vi "Aurora Tx Config.vi"(0 "6592R Resources":T3[](array[typedef]), 7 "FIFO Depth":u32=10240000 format="%#.6p", 11 "error in (no error)":errorcluster, 12 "tx config":T1={"rf enable 0"=FALSE, "rf config 0"={"antenna"="TX1", "frequency"=2000000000.0, "lo frequency"=-1.0, "level"=0.0}, "rf enable 1"=FALSE, "rf config 1"={"antenna"="TX1", "frequency"=2000000000.0, "lo frequency"=-1.0, "level"=0.0}, "transfer mode"=enum."Finite", "sample rate"=10000000.0, "start trigger"=enum."Immediate"} {"sample rate" format="%#.3pS/s"; "rf config 0"."level" format="%#_gdBm"; "rf config 0"."lo frequency" format="%#.3pHz"; "rf config 0"."frequency" format="%#.3pHz"; "rf config 1"."level" format="%#_gdBm"; "rf config 1"."lo frequency" format="%#.3pHz"; "rf config 1"."frequency" format="%#.3pHz"}) -> (4 "Ports used":bool[](array[boolean]), 6 "Refnum out":refnum<k20>[](array[refnum]), 8 "Actual FIFO Depths":u32[][](array[numeric]), 10 "2 Ports?":bool[](array[boolean]), 15 "error out":errorcluster)   [LabVIEW 2016]
uses:
  <vilib>/userdefined/Silver/nirio_resource_slv.ctl
  TypeDefs/Tx Config.ctl
  2954/SubVIs/Start Trigger.ctl
  6592R/SubVIs/Aurora Stream (NI 6592R) (Host).lvlib
panel:
  out "sFrontEndConfig_Complete":bool
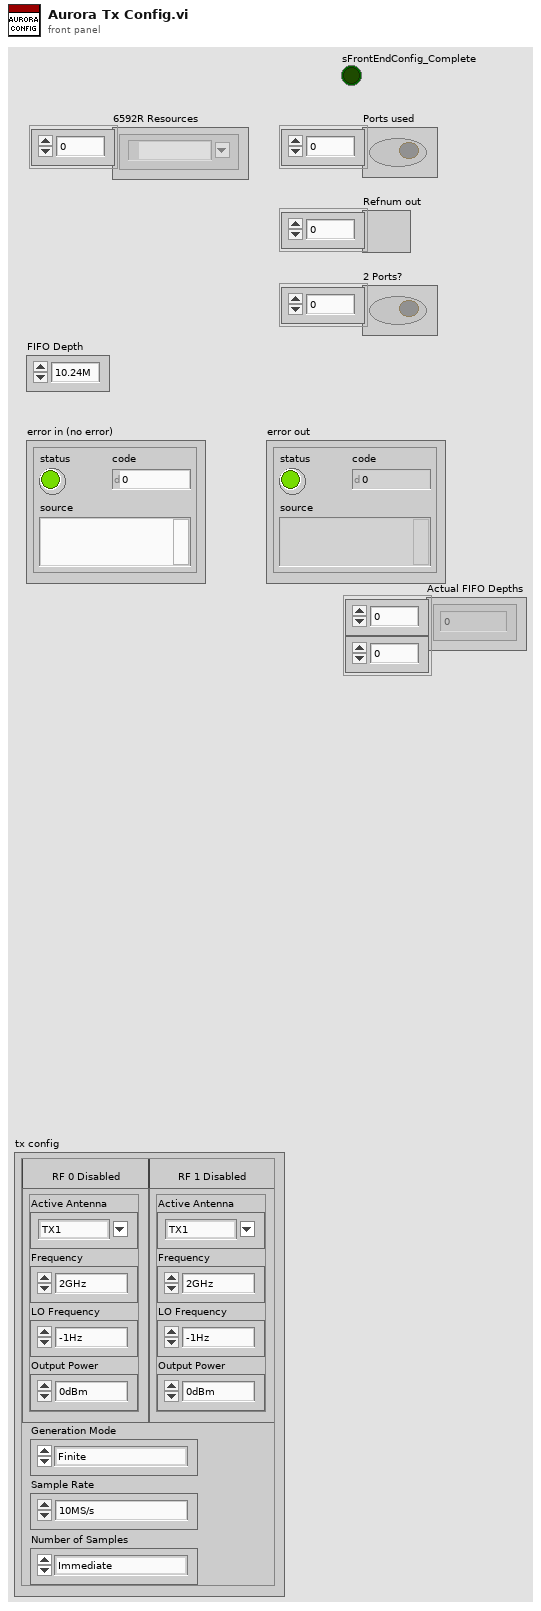
[diagram p1: front panel]
types:
  T1 = typedef "Tx Config.ctl" = cluster{"rf enable 0":bool, "rf config 0":cluster{"antenna":string, "frequency":dbl, "lo frequency":dbl, "level":dbl}, "rf enable 1":bool, "rf config 1":cluster{"antenna":string, "frequency":dbl, "lo frequency":dbl, "level":dbl}, "transfer mode":enum16{"Finite", "Continuous"}, "sample rate":dbl, "start trigger":T2}
  T2 = typedef "Start Trigger.ctl" = enum8{"Software", "Digital Edge", "Rx Start Trigger", "Tx Start Trigger", "Immediate", "Future Time Event"}
  T3 = typedef "nirio_resource_slv.ctl" = tag
  T4 = cluster{"Hard Error":bool, "Soft Error":bool, "Lane Up":bool, "Channel Up":bool, "Sys Reset":bool}
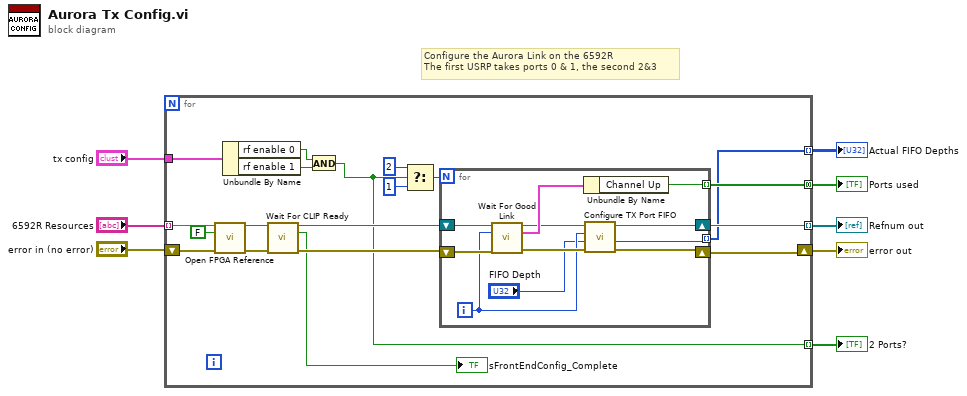
[diagram p0: block diagram]
diagram:
  # "Configure the Aurora Link on the 6592R\nThe first USRP takes ports 0 & 1, the second 2&3"
  n1 = for {
    tunnel: [w20] -> w5 mode=indexing
    tunnel: "6592R Resources" -> [w25] mode=indexing
    shift-right: [w21] -> w4
    shift-left: "error in (no error)" -> [w24]
    tunnel: [w17] -> w8 mode=concatenating
    tunnel: [w14] -> w3 mode=indexing
    tunnel: "tx config" -> [w13]
    tunnel: [w12] -> w1 mode=indexing
    n2 = call "Open FPGA Reference.vi"("FPGA Resource"=w25, "Rx?"=FALSE, "error in"=w24) -> ("FPGA VI Reference Out"=w26:refnum<k20>, "error out"=w27:errorcluster)  [unwired: 11 in]
    n3 = Unbundle By Name(w13) -> ("rf enable 0"=w11:bool, "rf enable 1"=w10:bool)
    n4 = call "Wait For CLIP Ready.vi"("Refnum in"=w26, "error in"=w27) -> ("Refnum out"=w23:refnum<k20>, "sFrontEndConfig_Complete"=→"sFrontEndConfig_Complete":bool, "error out"=w22:errorcluster)  [unwired: 11 in]
    n5 = And(x=w11, y=w10) -> (x .and. y?=w14:bool)
    n6 = Select(t=2, s=w14, f=1) -> (s? t:f=w15:i32)
    n7 = for {
      N: w15 -> [_]
      shift-right: [w31] -> w21
      shift-left: w22 -> [w38]
      shift-right: [w33] -> w20
      shift-left: w23 -> [w37]
      tunnel: [w35] -> w17 mode=indexing
      tunnel: [w30] -> w12 mode=indexing
      i -> [w29]
      n8 = call "Wait For Good Link.vi"("Refnum in"=w37, "Port"=w29, "error in"=w38) -> ("Refnum out"=w34:refnum<k20>, "Port Debug Info"=w36:T4, "error out"=w32:errorcluster)  [unwired: 10 in]
      n9 = Unbundle By Name(w36) -> ("Channel Up"=w35:bool)
      n10 = call "Configure TX Port FIFO.vi"("error in"=w32, "FIFO Depth"="FIFO Depth", "TX Port"=w29, "Refnum in"=w34) -> ("error out"=w31:errorcluster, "Actual Depth"=w30:u32, "Refnum out"=w33:refnum<k20>)  [unwired: 5 in]
    }
  }
  "2 Ports?" <- w3
  "Ports used" <- w8
  "Refnum out" <- w5
  "error out" <- w4
  "Actual FIFO Depths" <- w1
